vi "UHR-Fleezers Control (host) -Leonardo 04-2018 V3_greenctrl.vi"(0 "Tab Green FB":T5(tab)=enum."Trap Control (RF)") -> ()   [LabVIEW 2013] (continued)
  n84 = property on="2D or 1D Scan" class="Bool (strict)"("Val(Sgnl)"=w155) -> ()  [unwired: 2 in, 2 out]
  n85 = xnode "Read/Write Control"("FPGA VI Reference In"=w152, "error in"=w172, "ai count"="AI Count (ticks)", "Interlace ON/OFF"=w138, "Number Interlace Cycles"=w137, "Set 1"=w18, "Set 2"=w17, "Set 3"=w16, "FB On/Off Set 1"=w259, "FB On/Off Set 2"=w258, "Interlace Off Parameters"=w136, "FB Setpoint Set 1"=w250, "FB Setpoint Set 2"=w249, "FB Gains"="PID gains", "FB output range"=cluster{"output high":i16, "output low":i16} {"output high"=3000, "output low"=0} ("FB output range 1"), "Cycles per step"=w235, "Scan BD"=w247, "Number of scans"=w231, "Scan steps"=w236, "Scan freq.  increment"=w237, "AO1 (Y)"=w219, "AO2 (X)"=w218, "Scan freq.  increment (MCL)"=w212, "Scan steps (MCL)"=w211, "Cycles per step (MCL)"=w210, "Number of scans (MCL)"=w209, "MCL count"=w135, "Cont. Scan (MCL)"=w208, "MCL Scan Axis"=w202, "1D or 2D Scan?"=w155, "N of AI1 Int Acq Sets"=w192, "BD 1 Delay (ticks)"="Freq switch delay", "Amp switch delay"="Amp switch delay", "Swap F1 and F2"="Swap F1 and F2", "APD Acq Rate Count"=w160, "APD to FIFO"=FALSE, "APD Gate Operating Mode"="APD Gate", "APD Gate ON Count"="APD Gate ON Count", "APD Gate OFF Count"="APD Gate OFF Count", "Invert APD Gate"="Invert APD Gate", "DIO count 1 (ticks)"="DIO count 1 (ticks)", "DIO count 2 (ticks)"="DIO count 2 (ticks)", "DIO count 3 (ticks)"="DIO count 3 (ticks)", "APD 1 AO scale factor"="APD 1 AO Mult.", "APD 2 AO scale factor"="APD 2 AO Mult.", "Diff FB Measurement?"=w23, "Dynamic Force FB (Ronen)"=w22, "Negate Diff?"=w21, "Next trap write delay (ticks)"="Next trap write delay (ticks)", "Phase offset method"="Phase offset method", "Phase Trap 1"="Phase increment trap 1", "RF phase reset before cycles"="RF phase reset before cycles", "Phase Trap 2"="Phase increment trap 2") -> ("FPGA VI Reference Out"=w130:T20, "error out"=w132:errorcluster)  [unwired: 1 in]
  n86 = local read "Green Laser ON/Interlacing"() -> (w133:bool)
  n87 = local read "Green laser mode"() -> (w134:enum32{"Laser ON", "Laser OFF", "Interlace"})
  n88 = local read "GI Frequency, OFF count"() -> (w126:u32)
  n89 = local read "GI Frequency, ON count"() -> (w125:u32)
  n90 = Multiply(x="Current When FB OFF (%)", y=655.35) -> (x*y=w116:dbl)
  n91 = local read "Green FB Count"() -> (w124:u32)
  n92 = Multiply(x="Green FB Setpoint (mV)", y=3.2767) -> (x*y=w113:dbl)
  n93 = To Unsigned Word Integer(number=w116) -> (unsigned 16bit integer=w114:u16)
  n94 = local read "Invert GI"() -> (w128:bool)
  n95 = To Word Integer(number=w113) -> (16bit integer=w111:i16)
  n96 = case shown="True" w133 {
    tunnel: w134 -> [_ w294]
    tunnel: [enum32{"Laser ON", "Laser OFF", "Interlace"}."Laser OFF" ("Green laser mode") w294] -> w127
    frame False {
    }
    frame True {
    }
  }
  n97 = local read "Trap Pos. AI1 X Pre-scale"() -> (w82:u16)
  n98 = local read "Trap Pos FB Monitor\nT1 or T2"() -> (w89:bool)
  n99 = local read "Trap Pos FB Int Count"() -> (w79:u16)
  n100 = local read "Trap Pos FB Negate Action"() -> (w88:bool)
  n101 = local read "Trap Pos. FB Offset Factor"() -> (w87:i64)
  n102 = local read "Trap Pos. FB Mult Factor"() -> (w86:i64)
  n103 = local read "Trap Pos. FB Gains"() -> (w84:T11)
  n104 = local read "Trap Pos. FB Range"() -> (w85:T12)
  n105 = xnode "Read/Write Control"("FPGA VI Reference In"=w130, "error in"=w132, "Green interlace ON count 2"=w125, "Green interlace OFF count 2"=w126, "Invert GI 2"=w128, "Operating Mode 2"=w127, "Green FB Gains"="Green FB Gains", "Green FB Setpoint"=w111, "Green FB On/Off"="Green FB On/Off", "Current Out"=w114, "Green int current ON count adj"="Green int current ON count adj", "Green FB Count"=w124, "Operating Mode"=w127, "Green interlace OFF count"=w126, "Green interlace ON count"=w125, "Invert GI"=w128, "Trap Pos FB Monitor T1 or T2"=w89, "Trap Pos FB Negate Action"=w88, "Trap Pos. FB Offset Factor"=w87, "Trap Pos. FB Mult Factor"=w86, "Trap pos. FB Range"=w85, "Trap Pos. FB Gains"=w84, "Force feedback"=FALSE, "AI1 X Scale"=w82, "Trap Pos to FIFO"=TRUE, "Trap Pos FB Int Count"=w79) -> ("FPGA VI Reference Out"=w129:T20, "error out"=w131:errorcluster)
  n106 = xnode "Invoke Method"("FPGA VI Reference In"=w129, "error in"=w131, "Requested Depth"="Trap AI FIFO Depth") -> ("FPGA VI Reference Out"=w92:T20, "error out"=w91:errorcluster)  [unwired: 1 out]
  n107 = xnode "Invoke Method"("FPGA VI Reference In"=w92, "error in"=w91, "Requested Depth"="Trap Position FIFO Depth") -> ("FPGA VI Reference Out"=w6:T20, "error out"=w4:errorcluster)  [unwired: 1 out]
  n108 = xnode "Invoke Method"("FPGA VI Reference In"=w6, "error in"=w4, "Requested Depth"="APD FIFO Depth (requires restart)") -> ("FPGA VI Reference Out"=w5:T20, "error out"=w3:errorcluster)  [unwired: 1 out]
  n109 = flat-sequence {
    tunnel: w153 -> [w299]
    tunnel: [w299] -> w152
    tunnel: [w295] -> w39
    tunnel: [w298] -> w151
    tunnel: [w297] -> w149
    tunnel: [w296] -> w150
    frame #0 {
      w296 = T16 {"Minimum"=60.0, "Maximum"=90.0, "Increment"=1.0} ("Min Max Inc")
      w297 = T16 {"Minimum"=0.0, "Maximum"=75.0, "Increment"=1.0} ("Data Entry Limits")
      w295 = T16 {"Minimum"=60.0, "Maximum"=90.0, "Increment"=1.0} ("Min Max Inc")
      w298 = T16 {"Minimum"=0.0, "Maximum"=75.0, "Increment"=1.0} ("Data Entry Limits")
      n110 = property on="BD 2 Frequency 1 (MHz)" class="DigNum (strict)"("Data Range"=w296) -> ()  [unwired: 2 in, 2 out]
      n111 = property on="BD 2 Frequency 3 (MHz)" class="DigNum (strict)"("Data Range"=w296) -> ()  [unwired: 2 in, 2 out]
      n112 = property on="BD 2 Frequency 2 (MHz)" class="DigNum (strict)"("Data Range"=w296) -> ()  [unwired: 2 in, 2 out]
      n113 = property on="BD 1 Frequency 1 (MHz)" class="DigNum (strict)"("Data Range"=w295) -> ()  [unwired: 2 in, 2 out]
      n114 = property on="BD 1 Frequency 2 (MHz)" class="DigNum (strict)"("Data Range"=w295) -> ()  [unwired: 2 in, 2 out]
      n115 = property on="BD 1 Frequency 3 (MHz)" class="DigNum (strict)"("Data Range"=w295) -> ()  [unwired: 2 in, 2 out]
      n116 = property on="BD 2 Amplitude 1 (%)" class="DigNum (strict)"("Data Range"=w297) -> ()  [unwired: 2 in, 2 out]
      n117 = property on="BD 2 Amplitude 2 (%)" class="DigNum (strict)"("Data Range"=w297) -> ()  [unwired: 2 in, 2 out]
      n118 = property on="BD 2 Amplitude 3 (%)" class="DigNum (strict)"("Data Range"=w297) -> ()  [unwired: 2 in, 2 out]
      n119 = property on="BD 1 Amplitude 3 (%)" class="DigNum (strict)"("Data Range"=w298) -> ()  [unwired: 2 in, 2 out]
      n120 = property on="BD 1 Amplitude 2 (%)" class="DigNum (strict)"("Data Range"=w298) -> ()  [unwired: 2 in, 2 out]
      n121 = property on="BD 1 Amplitude 1 (%)" class="DigNum (strict)"("Data Range"=w298) -> ()  [unwired: 2 in, 2 out]
      "X RF Frequency Limits (MHz)" <- w295
      "X RF Amplitude Limits (%)" <- w298
      "Y RF Amplitude Limits (%)" <- w297
      "Y RF Frequency Limits (MHz)" <- w296
    }
  }
  n122 = xnode "Invoke Method"("FPGA VI Reference In"=w5, "error in"=w3) -> ("FPGA VI Reference Out"=w59:T20, "error out"=w58:errorcluster)  [unwired: 1 in]
  n123 = flat-sequence "Initial FPGA Loop Relative Phase Adjustment" {
    tunnel: "Initial Phase Adjustment (APD 2 Gate)" -> [w301]
    tunnel: "Initial Phase Adjustment (GI) 2" -> [w302]
    tunnel: "Initial Phase Adj. (MCL)" -> [w303]
    tunnel: w58 -> [w304]
    tunnel: w59 -> [w305]
    tunnel: "Initial Phase Adjustment (GI)" -> [w306]
    tunnel: "Initial Phase Adjustment (AI1)" -> [w307]
    tunnel: [w307] -> w68
    tunnel: [w306] -> w67
    tunnel: [w305] -> w66
    tunnel: [w304] -> w65
    tunnel: [w303] -> w64
    tunnel: [w302] -> w63
    tunnel: [w301] -> w62
    tunnel: [w319] -> w178
    tunnel: [w313] -> w176
    tunnel: "Initial Phase Adjustment (APD Acq)" -> [w312]
    tunnel: "Initial Phase Adjustment (APD 1 Gate)" -> [w311]
    tunnel: "Initial Phase Adjustment (Green FB)" -> [w310]
    tunnel: w68 -> [w318]
    tunnel: w67 -> [w317]
    tunnel: w66 -> [w316]
    tunnel: w65 -> [w315]
    tunnel: w64 -> [w314]
    tunnel: w63 -> [w309]
    tunnel: w62 -> [w308]
    tunnel: w178 -> [w321]
    tunnel: [w322] -> w177
    tunnel: w176 -> [w322]
    tunnel: [w321] -> w175
    tunnel: w177 -> [w325]
    tunnel: w175 -> [w324]
    tunnel: [w327] -> w174
    tunnel: [w326] -> w173
    tunnel: [w329] -> w57
    tunnel: [w330] -> w60
    tunnel: w174 -> [w330]
    tunnel: w173 -> [w329]
    frame #0 {
      n124 = Wait (ms)(milliseconds to wait=u32 1000) -> ()  [unwired: 1 out]
    }
    frame #1 {
      n125 = xnode "Read/Write Control"("FPGA VI Reference In"=w316, "error in"=w315, "Phase count adjustment"=w318, "Phase count adjustment (GI)"=w317, "Phase count adjustment (MCL)"=w314, "Phase Count Adjustment (APD Acq)"=w312, "Phase count adjustment (APD 1 Gate)"=w311, "Phase count adjustment (APD 2 Gate)"=w308, "Phase count adjustment (Green FB)"=w310, "Phase count adjustment (GI) 2"=w309) -> ("FPGA VI Reference Out"=w313:T20, "error out"=w319:errorcluster)
    }
    frame #2 {
      n126 = Wait (ms)(milliseconds to wait=u32 1000) -> ()  [unwired: 1 out]
    }
    frame #3 {
      w323 = TRUE
      n127 = xnode "Read/Write Control"("FPGA VI Reference In"=w325, "error in"=w324, "+ phase"=w323, "+ phase (GI)"=w323, "+ phase (MCL)"=w323, "+ phase (APD Acq)"=w323, "+ phase (APD 1 Gate)"=w323, "+ phase (APD 2 Gate)"=w323, "+ phase (Green FB)"=w323, "+ phase (GI) 2"=w323) -> ("FPGA VI Reference Out"=w326:T20, "error out"=w327:errorcluster)
    }
    frame #4 {
      n128 = Wait (ms)(milliseconds to wait=u32 1000) -> ()  [unwired: 1 out]
    }
  }
  n129 = Unbundle By Name(w39) -> ("Minimum"=w38:dbl, "Maximum"=w37:dbl)
  n130 = local read "Phase adj. (Green FB)"() -> (w147:i16)
  n131 = local read "Phase adj. (GI) 2"() -> (w117:i16)
  n132 = local read "Phase adjust (MCL)"() -> (w203:i16)
  n133 = local read "Phase adj. (AI1)"() -> (w205:i16)
  n134 = local read "Phase adj. (GI)"() -> (w204:i16)
  n135 = Multiply(x=w38, y=w36) -> (x*y=w34:dbl)
  n136 = Multiply(x=w37, y=w36) -> (x*y=w35:dbl)
  n137 = Multiply(x=49152000.0, y=6.0) -> (x*y=w28:dbl)
  n138 = Scale By Power Of 2(n=w33, x=w34) -> (x*2^n=w30:dbl)
  n139 = Scale By Power Of 2(n=w33, x=w35) -> (x*2^n=w29:dbl)
  n140 = xnode "Read/Write Control"("FPGA VI Reference In"=w57, "error in"=w60, "Phase count adjustment"=w205, "Phase count adjustment (GI)"=w204, "Phase count adjustment (MCL)"=w203, "Phase Count Adjustment (APD Acq)"="Phase Adj. (APD Acq)", "Phase count adjustment (APD 1 Gate)"="Phase Adj. (APD 1 Gate)", "Phase count adjustment (APD 2 Gate)"="Phase Adj. (APD 2 Gate)", "Phase count adjustment (Green FB)"=w147, "Phase count adjustment (GI) 2"=w117) -> ("FPGA VI Reference Out"=w14:T20, "error out"=w13:errorcluster)
  n141 = Divide(x=w29, y=w28) -> (x/y=w26:dbl)
  n142 = Divide(x=w30, y=w28) -> (x/y=w27:dbl)
  n143 = To Unsigned Quad Integer(1:w27) -> (0:w25:u64)
  n144 = To Unsigned Quad Integer(1:w26) -> (0:w24:u64)
  n145 = xnode "Read/Write Control"("FPGA VI Reference In"=w14, "FB Min frequency"=w25, "FB Max Frequency"=w24) -> ()  [unwired: 1 in, 2 out]
  n146 = call "set RF board frequency - interlace.vi"("Board 2 Frequency Limits"=w150, "Board 1 Frequency Limits"=w39, "error in"=w13, "FPGA VI Reference In"=w14, "Board 2 Frequency 3 (MHz)"="BD 2 Frequency 3 (MHz)", "Board 1 Frequency 3 (MHz)"="BD 1 Frequency 3 (MHz)", "Board 2 Frequency 2 (MHz)"="BD 2 Frequency 2 (MHz)", "Board 2 Frequency 1 (MHz)"="BD 2 Frequency 1 (MHz)", "Board 1 Frequency 2 (MHz)"="BD 1 Frequency 2 (MHz)", "Board 1 Frequency 1  (MHz)"="BD 1 Frequency 1 (MHz)") -> ("error out"=w270:errorcluster, "FPGA VI Reference Out"=w271:T20)
  n147 = call "set RF board amplitude - interlace.vi"("Board 2 Amplitude Limits"=w149, "Board 1 Amplitude Limits"=w151, "error in"=w270, "FPGA VI Reference In"=w271, "Board 2 Amplitude 3 (%)"="BD 2 Amplitude 3 (%)", "Board 1 Amplitude 3 (%)"="BD 1 Amplitude 3 (%)", "Board 2 Amplitude 2 (%)"="BD 2 Amplitude 2 (%)", "Board 2 Amplitude 1 (%)"="BD 2 Amplitude 1 (%)", "Board 1 Amplitude 2 (%)"="BD 1 Amplitude 2 (%)", "Board 1 Amplitude 1 (%)"="BD 1 Amplitude 1 (%)") -> ("error out"=w55:errorcluster, "FPGA VI Reference Out"=w56:T20)
  n148 = flat-sequence {
    tunnel: w56 -> [w332]
    tunnel: w55 -> [w331]
    tunnel: [w332] -> w263
    tunnel: [w331] -> w262
    tunnel: [w340] -> w261
    tunnel: w263 -> [w340]
    tunnel: [w339] -> w260
    tunnel: w262 -> [w339]
    tunnel: w261 -> [w343]
    tunnel: w260 -> [w342]
    tunnel: [w343] -> w51
    tunnel: [w342] -> w50
    tunnel: [w349] -> w76
    tunnel: [w353] -> w61
    tunnel: w51 -> [w353]
    tunnel: w50 -> [w348]
    frame #0 {
      n149 = local read "Trap 1 (ON/OFF)"() -> (w333:bool)
      n150 = local write "Saving..."(FALSE ("Saving Data")) -> ()
      n151 = local write "Stop All"(FALSE ("Stop All")) -> ()
      n152 = local write "Index"(1.0 ("Index")) -> ()
      n153 = property on="Trap 1 ON" class="Bool (strict)"("Value"=w333) -> ()  [unwired: 2 in, 2 out]
      "Manipulating Trap" <- FALSE ("Manipulating Trap")
    }
    frame #1 {
      n154 = local read "Trap 2 (ON/OFF)"() -> (w338:bool)
      n155 = Wait (ms)(milliseconds to wait=u32 50) -> ()  [unwired: 1 out]
      n156 = property on="Trap 2 ON" class="Bool (strict)"("Val(Sgnl)"=w338) -> ()  [unwired: 2 in, 2 out]
    }
    frame #2 {
      n157 = local read "Scan Range (nm)"() -> (w344:dbl)
      n158 = call "Update messages.vi"("Message to add"="UHR-Fleezers ready.", "Old message string"="") -> ("New message string"=w347:string)
      n159 = local write "Messages"(w347) -> ()
      n160 = property on="Scan Range (nm)" class="DigNum (strict)"("Val(Sgnl)"=w344) -> ()  [unwired: 2 in, 2 out]
    }
    frame #3 {
      n161 = call "hamilton_controller.vi"("error in"=w348, "action"=T21."CONNECT") -> ("error out"=w350:errorcluster)  [unwired: 9 in]
      n162 = call "hamilton_controller.vi"("error in"=w350, "action"=T21."INITIALIZE VALVES") -> ("error out"=w349:errorcluster)  [unwired: 9 in]
    }
  }
  n163 = Subtract(x="BD 1 Frequency 1 (MHz)", y="BD 1 Frequency 2 (MHz)") -> (x-y=w191:dbl)
  n164 = Subtract(x="BD 2 Frequency 1 (MHz)", y="BD 2 Frequency 2 (MHz)") -> (x-y=w190:dbl)
  n165 = Square(x=w190) -> (x^2=w188:dbl)
  n166 = Square(x=w191) -> (x^2=w189:dbl)
  n167 = Add(x=w189, y=w188) -> (x+y=w187:dbl)
  n168 = Square Root(x=w187) -> (sqrt(x)=w186:dbl)
  n169 = local write "Trap Delta (MHz)"(w186) -> ()
  n170 = call "IMAQ Create"("Image Name"="APD 1 Image", "Image Type"=w98) -> ("New Image"=w97:T3)  [unwired: 3 in, 1 out]
  n171 = call "IMAQ Create"("Image Name"="APD 2 Image", "Image Type"=w98) -> ("New Image"=w96:T3)  [unwired: 3 in, 1 out]
  n172 = call "IMAQ Create"("Image Name"="Det. X Image", "Image Type"=w98) -> ("New Image"=w95:T3)  [unwired: 3 in, 1 out]
  n173 = call "IMAQ Create"("Image Name"="Det. Y Image", "Image Type"=w98) -> ("New Image"=w94:T3)  [unwired: 3 in, 1 out]
  n174 = Bundle("New Image"=w97, "New Image"=w96, "New Image"=w95, "New Image"=w94) -> (w93:T22)  [unwired: 1 in]
  n175 = Current VI's Path() -> (path=w40:path)
  n176 = Concatenate Strings("N.D.", "\r\n") -> (w44:string)
  n177 = Strip Path(path=w40) -> (stripped path=w41:path)  [unwired: 1 out]
  n178 = Initialize Array(w44, 4, 3) -> (w47:string[][])
  n179 = Build Path(base path=w41, name or relative path="Locations.txt") -> (appended path=→"Location path":path)
  n180 = local write "Location Matrix"(w47) -> ()
  n181 = while {
    stop <- w354 stop-if-true
    n182 = event shown="[0] Timeout" {
      selector: _ -> [_ _ _ _ _ _ _ _ _]
      dyn-events: _ -> [_ _ _ _ _ _ _ _ _]
      timeout: 10 -> [_ _ _ _ _ _ _ _ _]
      tunnel: [FALSE _ _ _ _ _ _ _ TRUE] -> w354
      event Timeout {
        # "Change the trajectory mode to Jog"
        # "Query and display stage positions"
        # "Setting ESP300 left and right limits for Z-axis, input in mm"
        # "Display Selected Location"
        n183 = event-data() -> ()  [unwired: 1 in, 2 out]
        n184 = local read "Capture Locations"() -> (w379:i32)
        n185 = local read "Location Matrix"() -> (w380:string[][])
        n186 = Concatenate Strings("1TP;\n2TP;\n3TP;\n1MD?;\n2MD?;\n3MD?" ("Substring"), "\r") -> (w363:string)
        n187 = local read "ESP Port"() -> (w366:refnum<visa-resource-name>)
        n188 = Index Array(array=w380, index (row)=w379) -> (element=w378:string[])  [unwired: 1 in]
        n189 = local read "ESP Port"() -> (w375:refnum<visa-resource-name>)
        n190 = VISA Write(VISA resource name=w366, write buffer=w363, error in (no error)="error in") -> (VISA resource name out=w364:refnum<visa-resource-name>, error out=w362:errorcluster)  [unwired: 1 out]
        n191 = Concatenate Strings("3SL" ("Substring"), "ESP ZL-Limit", ";3SR", "ESP ZR-Limit", "\r") -> (w374:string)
        n192 = Array To Cluster(array=w378) -> (cluster=w377:T23)
        n193 = case shown="True" TRUE ("Case Constant\n(See Context Help)") {
          tunnel: w364 -> [_ w418]
          tunnel: w362 -> [w399 w417]
          tunnel: [w399 w401] -> w368
          frame False {
          }
          frame True {
            w411 = u16 10 items=["1.0"=10, "1.5"=15, "2.0"=20] ("Serial Settings:Stop Bits")
            w412 = u16 0 items=["None", "Odd", "Even", "Mark", "Space"] ("Serial Settings:Parity")
            n194 = property class="Instr"(reference=w418, error in=w417, "Baud"=u32 921600 ("Serial Settings:Baud Rate"), "Data Bits"=u16 8 ("Serial Settings:Data Bits"), "Parity"=w412, "Stop Bits"=w411) -> (reference out=w416:refnum<visa-resource-name>, error out=w415:errorcluster, "Bytes at Port"=w400:u32)
            n195 = Wait (ms)(milliseconds to wait=u32 10) -> ()  [unwired: 1 out]
            n196 = VISA Read(VISA resource name=w416, byte count=w400, error in (no error)=w415) -> (VISA resource name out=w424:refnum<visa-resource-name>, read buffer=→"X Pos":string, error out=w425:errorcluster)  [unwired: 1 out]
            n197 = VISA Read(VISA resource name=w424, byte count=w400, error in (no error)=w425) -> (VISA resource name out=w422:refnum<visa-resource-name>, read buffer=→"Y Pos":string, error out=w423:errorcluster)  [unwired: 1 out]
            n198 = VISA Read(VISA resource name=w422, byte count=w400, error in (no error)=w423) -> (VISA resource name out=w410:refnum<visa-resource-name>, read buffer=→"Z Pos Pos":string, error out=w409:errorcluster)  [unwired: 1 out]
            n199 = VISA Read(VISA resource name=w410, byte count=w400, error in (no error)=w409) -> (VISA resource name out=w406:refnum<visa-resource-name>, read buffer=→"X Motion":string, error out=w407:errorcluster)  [unwired: 1 out]
            n200 = VISA Read(VISA resource name=w406, byte count=w400, error in (no error)=w407) -> (VISA resource name out=w405:refnum<visa-resource-name>, read buffer=→"Y Motion":string, error out=w403:errorcluster)  [unwired: 1 out]
            n201 = VISA Read(VISA resource name=w405, byte count=w400, error in (no error)=w403) -> (read buffer=→"Z motion":string, error out=w401:errorcluster)  [unwired: 2 out]
          }
        }
        "error out" <- w368
        n202 = VISA Write(VISA resource name=w375, write buffer=w374) -> ()  [unwired: 1 in, 3 out]
        n203 = local write item#483(w377) -> ()
        n204 = disable-structure shown="Disabled" {
          frame Disabled {
            # "Change Low Jog Velocity"
            # "Change High Jog Velocity"
            n205 = Concatenate Strings("1JH" ("Substring"), "Axis 1", "2JH" ("Substring"), "Axis 2", "3JH" ("Substring"), "Axis 3", "\r") -> (w398:string)
            n206 = local read "ESP Port"() -> (w397:refnum<visa-resource-name>)
            n207 = VISA Write(VISA resource name=w397, write buffer=w398) -> ()  [unwired: 1 in, 3 out]
            n208 = Concatenate Strings("1JW" ("Substring"), "Axis 1", "2JW" ("Substring"), "Axis 2", "3JW" ("Substring"), "Axis 3", "\r") -> (w389:string)
            n209 = local read "ESP Port"() -> (w388:refnum<visa-resource-name>)
            n210 = VISA Write(VISA resource name=w388, write buffer=w389) -> ()  [unwired: 1 in, 3 out]
          }
          frame Enabled {
          }
        }
        n211 = local read "ESP Port"() -> (w356:refnum<visa-resource-name>)
        n212 = Concatenate Strings("1TJ3;\n2TJ3;\n3TJ3" ("Substring"), "\r") -> (w357:string)
        n213 = VISA Write(VISA resource name=w356, write buffer=w357) -> ()  [unwired: 1 in, 3 out]
      }
      event "Goto Top (F6)": Value Change {
        n214 = event-data() -> ()  [unwired: 1 in, 5 out]
        n215 = stacked-sequence {
          frame #0 {
            # "stop motions of all axes before going to avoid reversing of direction"
            n216 = local read "ESP Port"() -> (w430:refnum<visa-resource-name>)
            n217 = Concatenate Strings("ST" ("Substring"), "\r") -> (w427:string)
            n218 = VISA Write(VISA resource name=w430, write buffer=w427) -> ()  [unwired: 1 in, 3 out]
          }
          frame #1 {
            n219 = Wait (ms)(milliseconds to wait=u32 50) -> ()  [unwired: 1 out]
          }
          frame #2 {
            # "Change the trajectory mode to Trapezoidal"
            n220 = local read "ESP Port"() -> (w435:refnum<visa-resource-name>)
            n221 = Concatenate Strings("1TJ1;\n2TJ1;\n3TJ1" ("Substring"), "\r") -> (w432:string)
            n222 = VISA Write(VISA resource name=w435, write buffer=w432) -> ()  [unwired: 1 in, 3 out]
          }
          frame #3 {
            # "Go to Top Dispensor"
            n223 = local read "Location Matrix"() -> (w447:string[][])
            n224 = Index Array(array=w447, index (row)=0) -> (element=w443:string[])  [unwired: 1 in]
            n225 = Decimate 1D Array(w443) -> (w441:string[], w439:string[], w437:string[])
            n226 = local read "ESP Port"() -> (w444:refnum<visa-resource-name>)
            n227 = Concatenate Strings("1PA" ("Substring"), w441, "2PA" ("Substring"), w439, "3PA" ("Substring"), w437, "\r") -> (w445:string)
            n228 = VISA Write(VISA resource name=w444, write buffer=w445) -> ()  [unwired: 1 in, 3 out]
          }
          frame #4 {
            n229 = Wait (ms)(milliseconds to wait=u32 100) -> ()  [unwired: 1 out]
          }
          frame #5 {
            # "Change the trajectory mode to Jog"
            n230 = local read "ESP Port"() -> (w452:refnum<visa-resource-name>)
            n231 = Concatenate Strings("1TJ3;\n2TJ3;\n3TJ3" ("Substring"), "\r") -> (w449:string)
            n232 = VISA Write(VISA resource name=w452, write buffer=w449) -> ()  [unwired: 1 in, 3 out]
          }
        }
      }
      event "Goto Exp (F8)": Value Change {
        n233 = event-data() -> ()  [unwired: 1 in, 5 out]
        n234 = stacked-sequence {
          frame #0 {
            # "stop motions of all axes before going to avoid reversing of direction"
            n235 = local read "ESP Port"() -> (w456:refnum<visa-resource-name>)
            n236 = Concatenate Strings("ST" ("Substring"), "\r") -> (w453:string)
            n237 = VISA Write(VISA resource name=w456, write buffer=w453) -> ()  [unwired: 1 in, 3 out]
          }
          frame #1 {
            n238 = Wait (ms)(milliseconds to wait=u32 50) -> ()  [unwired: 1 out]
          }
          frame #2 {
            # "Change the trajectory mode to Trapezoidal"
            n239 = local read "ESP Port"() -> (w461:refnum<visa-resource-name>)
            n240 = Concatenate Strings("1TJ1;\n2TJ1;\n3TJ1" ("Substring"), "\r") -> (w458:string)
            n241 = VISA Write(VISA resource name=w461, write buffer=w458) -> ()  [unwired: 1 in, 3 out]
          }
          frame #3 {
            # "Go to Experimental"
            n242 = local read "Location Matrix"() -> (w473:string[][])
            n243 = Index Array(array=w473, index (row)=2) -> (element=w469:string[])  [unwired: 1 in]
            n244 = Decimate 1D Array(w469) -> (w467:string[], w465:string[], w463:string[])
            n245 = Concatenate Strings("1PA" ("Substring"), w467, "2PA" ("Substring"), w465, "3PA" ("Substring"), w463, "\r") -> (w471:string)
            n246 = local read "ESP Port"() -> (w470:refnum<visa-resource-name>)
            n247 = VISA Write(VISA resource name=w470, write buffer=w471) -> ()  [unwired: 1 in, 3 out]
          }
          frame #4 {
            n248 = Wait (ms)(milliseconds to wait=u32 200) -> ()  [unwired: 1 out]
          }
          frame #5 {
            # "Change the trajectory mode to Jog"
            n249 = local read "ESP Port"() -> (w475:refnum<visa-resource-name>)
            n250 = Concatenate Strings("1TJ3;\n2TJ3;\n3TJ3" ("Substring"), "\r") -> (w478:string)
            n251 = VISA Write(VISA resource name=w475, write buffer=w478) -> ()  [unwired: 1 in, 3 out]
          }
        }
      }
      event "Goto Bottom (F7)": Value Change {
        n252 = event-data() -> ()  [unwired: 1 in, 5 out]
        n253 = stacked-sequence {
          frame #0 {
            # "stop motions of all axes before going to avoid reversing of direction"
            n254 = local read "ESP Port"() -> (w482:refnum<visa-resource-name>)
            n255 = Concatenate Strings("ST" ("Substring"), "\r") -> (w479:string)
            n256 = VISA Write(VISA resource name=w482, write buffer=w479) -> ()  [unwired: 1 in, 3 out]
          }
          frame #1 {
            n257 = Wait (ms)(milliseconds to wait=u32 50) -> ()  [unwired: 1 out]
          }
          frame #2 {
            # "Change the trajectory mode to Trapezoidal"
            n258 = local read "ESP Port"() -> (w487:refnum<visa-resource-name>)
            n259 = Concatenate Strings("1TJ1;\n2TJ1;\n3TJ1" ("Substring"), "\r") -> (w484:string)
            n260 = VISA Write(VISA resource name=w487, write buffer=w484) -> ()  [unwired: 1 in, 3 out]
          }
          frame #3 {
            # "Go to Bottom Dispensor"
            n261 = local read "Location Matrix"() -> (w499:string[][])
            n262 = Index Array(array=w499, index (row)=1) -> (element=w495:string[])  [unwired: 1 in]
            n263 = Decimate 1D Array(w495) -> (w493:string[], w491:string[], w489:string[])
            n264 = Concatenate Strings("1PA" ("Substring"), w493, "2PA" ("Substring"), w491, "3PA" ("Substring"), w489, "\r") -> (w497:string)
            n265 = local read "ESP Port"() -> (w496:refnum<visa-resource-name>)
            n266 = VISA Write(VISA resource name=w496, write buffer=w497) -> ()  [unwired: 1 in, 3 out]
          }
          frame #4 {
            n267 = Wait (ms)(milliseconds to wait=u32 200) -> ()  [unwired: 1 out]
          }
          frame #5 {
            # "Change the trajectory mode to Jog"
            n268 = local read "ESP Port"() -> (w501:refnum<visa-resource-name>)
            n269 = Concatenate Strings("1TJ3;\n2TJ3;\n3TJ3" ("Substring"), "\r") -> (w504:string)
            n270 = VISA Write(VISA resource name=w501, write buffer=w504) -> ()  [unwired: 1 in, 3 out]
          }
        }
      }
      event "Capture": Value Change {
        n271 = event-data() -> ()  [unwired: 1 in, 5 out]
        n272 = local read "Capture Locations"() -> (w505:i32)
        n273 = local read "Z Pos Pos"() -> (w506:string)
        n274 = local read "X Pos"() -> (w508:string)
        n275 = local read "Y Pos"() -> (w507:string)
        n276 = case shown="1" w505 {
          selector: w505 -> [w512 w519 w526 w533]
          tunnel: w508 -> [w515 w522 w529 w536]
          tunnel: w507 -> [w514 w521 w528 w535]
          tunnel: w506 -> [w513 w520 w527 w534]
          frame 0, Default {
            # "Capture Top Dispensor Location"
            n277 = local read "Location Matrix"() -> (w511:string[][])
            n278 = Build Array(w515, w514, w513) -> (w510:string[])
            n279 = Replace Array Subset(array=w511, new element=w510, index (row)=w512) -> (w509:string[][])  [unwired: 1 in]
            n280 = local write "Location Matrix"(w509) -> ()
          }
          frame 1 {
            # "Capture Bottom Dispensor Location"
            n281 = local read "Location Matrix"() -> (w518:string[][])
            n282 = Build Array(w522, w521, w520) -> (w517:string[])
            n283 = Replace Array Subset(array=w518, new element=w517, index (row)=w519) -> (w516:string[][])  [unwired: 1 in]
            n284 = local write "Location Matrix"(w516) -> ()
          }
          frame 2 {
            # "Capture Experimental Region Location"
            n285 = local read "Location Matrix"() -> (w525:string[][])
            n286 = Build Array(w529, w528, w527) -> (w524:string[])
            n287 = Replace Array Subset(array=w525, new element=w524, index (row)=w526) -> (w523:string[][])  [unwired: 1 in]
            n288 = local write "Location Matrix"(w523) -> ()
          }
          frame 3 {
            # "Capture Other Location"
            n289 = local read "Location Matrix"() -> (w532:string[][])
            n290 = Build Array(w536, w535, w534) -> (w531:string[])
            n291 = Replace Array Subset(array=w532, new element=w531, index (row)=w533) -> (w530:string[][])  [unwired: 1 in]
            n292 = local write "Location Matrix"(w530) -> ()
          }
        }
      }
      event "Save": Value Change {
        # "reshape Location Matrix to 1-D array to write"
        n293 = event-data() -> ()  [unwired: 1 in, 5 out]
        n294 = local read "Location Matrix"() -> (w540:string[][])
        n295 = local read "Location path"() -> (w537:path)
        n296 = Reshape Array(w540, 12) -> (w538:string[])
        n297 = Write to Text File(file (use dialog)=w537, text=w538) -> ()  [unwired: 2 in, 3 out]
      }
      event "VISA Clear": Value Change {
        n298 = event-data() -> ()  [unwired: 1 in, 5 out]
        n299 = local read "ESP Port"() -> (w541:refnum<visa-resource-name>)
        n300 = VISA Clear(VISA resource name=w541) -> ()  [unwired: 1 in, 2 out]
      }
      event "Activate Joystick": Value Change {
        # "Change the trajectory mode to Jog"
        n301 = event-data() -> ()  [unwired: 1 in, 5 out]
        n302 = disable-structure shown="Disabled" {
          frame Disabled {
            n303 = case shown="True" "Activate Joystick" {
              frame False {
              }
              frame True {
                # "Change the trajectory mode to Jog"
                n304 = local read "ESP Port"() -> (w550:refnum<visa-resource-name>)
                n305 = Concatenate Strings("1TJ3;\n2TJ3;\n3TJ3" ("Substring"), "\r") -> (w547:string)
                n306 = VISA Write(VISA resource name=w550, write buffer=w547) -> ()  [unwired: 1 in, 3 out]
              }
            }
          }
          frame Enabled {
          }
        }
        n307 = local read "ESP Port"() -> (w542:refnum<visa-resource-name>)
        n308 = Concatenate Strings("1TJ3;\n2TJ3;\n3TJ3" ("Substring"), "\r") -> (w545:string)
        n309 = VISA Write(VISA resource name=w542, write buffer=w545) -> ()  [unwired: 1 in, 3 out]
      }
      event "Stop All": Mouse Down {
        n310 = event-data() -> ()  [unwired: 1 in, 5 out]
      }
    }
  }
  n311 = disable-structure shown="Disabled" {
    disable-tunnel: w61 -> [w580 _]
    frame Disabled {
      w575 = T17 0 items=["Grayscale (U8)", "Grayscale (I16)", "Grayscale (SGL)", "Complex (CSG)", "RGB (U32)", "HSL (U32)", "RGB (U64)", "Grayscale (U16)"] ("Image Type")
      n312 = call <vilib>:"IMAQ Init.vi"("Interface Name"="img0") -> ("error out"=w577:errorcluster, "IMAQ Session Out"=w579:refnum<k11>)  [unwired: 9 in]
      n313 = call <vilib>:"IMAQ Grab Setup.vi"("error in (no error)"=w577, "IMAQ Session In"=w579) -> ("error out"=w573:errorcluster, "IMAQ Session Out"=w574:refnum<k11>)  [unwired: 8 in]
      n314 = call "IMAQ Create"("Image Name"="untitled", "Image Type"=w575) -> ("New Image"=w572:T3)  [unwired: 3 in, 1 out]
      n315 = call <vilib>:"Application Directory.vi"() -> ("Application Directory"=w559:path)
      n316 = Build Path(base path=w559, name or relative path="_trap_screen_positions") -> (appended path=w567:path)
      n317 = Open/Create/Replace File(file path (use dialog)=w567, operation (0:open)=T24."open or create", access (0:read/write)=enum16{"read/write", "read-only", "write-only"}."read/write") -> (refnum out=w569:refnum<file>)  [unwired: 3 in, 2 out]
      n318 = local read "Trap Sets"() -> (w561:u32)
      n319 = for "Load trap positions on video screen from file." {
        N: w561 -> [_]
        tunnel: [w587] -> w562
        tunnel: w569 -> [w586]
        tunnel: [w583] -> w558 mode=indexing
        w585 = 4
        n320 = for {
          N: w585 -> [_]
          tunnel: [w591] -> w587
          tunnel: w586 -> [w590]
          tunnel: w585 -> [w589]
          tunnel: [w588] -> w584 mode=indexing
          n321 = Read from Binary File(5:w589, 11:w590) -> (2:w588:i32, 3:w591:refnum<file>)  [unwired: 4 in, 2 out]
        }
        n322 = Array To Cluster(array=w584) -> (cluster=w583:T28)
      }
      n323 = node-c288() -> (w582:T25)  [unwired: 4 in]
      n324 = timed-loop "acquire video and stage position" {
        timing: w582 -> [_]
        timing-out: [_] -> w581
        tunnel: w574 -> [w610]
        tunnel: w573 -> [w609]
        tunnel: w572 -> [w608]
        tunnel: [w607] -> w554
        tunnel: [w604] -> w555
        tunnel: [w605] -> w553
        tunnel: w580 -> [_]
        shift-right: [w601] -> w571
        shift-left: w558 -> [w602]
        tunnel: w561 -> [w599]
        stop <- w606 stop-if-true
        n325 = node-c288() -> ()  [unwired: 1 in, 1 out]
        n326 = event shown="[1] \"Stop All\": Value Change" {
          selector: _ -> [_ _ _ _]
          dyn-events: _ -> [_ _ _ _]
          timeout: 10 -> [_ _ _ _]
          tunnel: w610 -> [w621 w636 w645 w664]
          tunnel: w609 -> [w620 w638 w643 w666]
          tunnel: w608 -> [w619 w637 w644 w665]
          tunnel: [w618 w636 w645 w664] -> w607
          tunnel: [w611 w640 FALSE FALSE] -> w606
          tunnel: [w615 w638 w643 w666] -> w605
          tunnel: [w614 w637 w644 w665] -> w604
          tunnel: "radius" -> [_ _ w650 _]
          tunnel: w602 -> [w612 w639 w648 _]
          tunnel: [w612 w639 w649 cluster{i32, i32, i32, i32}[] []] -> w601
          tunnel: w599 -> [_ _ w641 _]
          event Timeout {
            n327 = event-data() -> ()  [unwired: 1 in, 2 out]
            n328 = call <vilib>:"IMAQ Grab Acquire.vi"("error in (no error)"=w620, "Image In"=w619, "IMAQ Session In"=w621) -> ("error out"=w616:errorcluster, "Image Out"=w617:T3, "IMAQ Session Out"=w618:refnum<k11>)  [unwired: 5 in, 1 out]
            n329 = case shown="True" "trap\nmarkers?" {
              tunnel: w612 -> [_ w629]
              tunnel: w617 -> [w623 w628]
              tunnel: w616 -> [w622 w627]
              tunnel: [w622 w626] -> w615
              tunnel: [w623 w624] -> w614
              frame False {
              }
              frame True {
                n330 = for {
                  tunnel: w629 -> [w635] mode=indexing
                  shift-right: [w633] -> w624
                  shift-left: w628 -> [w634]
                  tunnel: w627 -> [w632]
                  tunnel: [w631] -> w626
                  tunnel: u32 16711680 ("Color") -> [w630]
                  n331 = call "IMAQ Overlay Oval"("Color"=w630, "error in (no error)"=w632, "Bounding Rectangle"=w635, "Image"=w634) -> ("error out"=w631:errorcluster, "Image Out"=w633:T3)  [unwired: 6 in]
                }
              }
            }
            "Primary Video Display" <- w614
            n332 = Unbundle By Name(w616) -> ("status"=w611:bool)
          }
          event "Stop All": Value Change {
            n333 = event-data() -> ()  [unwired: 1 in, 5 out]
            n334 = local read "Stop All"() -> (w640:bool)
          }
          event "Primary Video Display": Mouse Down {
            n335 = event-data() -> ()  [unwired: 1 in, 7 out]
            n336 = Array Size(array=w648) -> (size(s)=w647:i32)
            n337 = Less?(x=w647, y=w641) -> (x < y?=w646:bool)
            n338 = case shown="True" w646 {
              tunnel: w650 -> [_ w660]
              tunnel: w648 -> [w651 w654]
              tunnel: [w651 w653] -> w649
              frame False {
              }
              frame True {
                n339 = property on="Primary Video Display" class="ImageControl"() -> ("Last Mouse Position"=w652:cluster{"X":i32, "Y":i32})  [unwired: 2 in, 2 out]
                n340 = Unbundle By Name(w652) -> ("X"=w662:i32, "Y"=w661:i32)
                n341 = Add(x=w661, y=w660) -> (x+y=w658:i32)
                n342 = Subtract(x=w661, y=w660) -> (x-y=w656:i32)
                n343 = Add(x=w662, y=w660) -> (x+y=w657:i32)
                n344 = Subtract(x=w662, y=w660) -> (x-y=w659:i32)
                n345 = Bundle(w659, w658, w657, w656) -> (w655:cluster{i32, i32, i32, i32})  [unwired: 1 in]
                n346 = Build Array (concatenate)(w654, w655) -> (w653:T29)
              }
            }
          }
          event "clear markers": Value Change {
            n347 = event-data() -> ()  [unwired: 1 in, 5 out]
          }
        }
        n348 = node-c288() -> ()  [unwired: 1 in, 1 out]
      }
      n349 = node-c288(w581) -> ()  [unwired: 1 out]
      n350 = Set File Position(offset (in bytes) (0)=i64 0, refnum=w562, from (0:start)=enum16{"start", "end", "current"}."start") -> (refnum out=w563:refnum<file>)  [unwired: 1 in, 1 out]
      n351 = for "Write trap positions to file so they can be remembered\nwhen program is removed from memory" {
        tunnel: w571 -> [w595] mode=indexing
        tunnel: [w593] -> w570
        tunnel: w563 -> [w592]
        n352 = Cluster To Array(cluster=w595) -> (array=w594:i32[])
        n353 = for {
          tunnel: w594 -> [w598] mode=indexing
          tunnel: [w597] -> w593
          tunnel: w592 -> [w596]
          n354 = Write to Binary File(file (use dialog)=w596, data=w598) -> (refnum out=w597:refnum<file>)  [unwired: 4 in, 2 out]
        }
      }
      n355 = Close File(refnum=w570) -> ()  [unwired: 1 in, 2 out]
      n356 = call "IMAQ Dispose"("Image"=w555, "error in (no error)"=w553) -> ("error out"=w552:errorcluster)  [unwired: 4 in]
      n357 = call <vilib>:"IMAQ Stop.vi"("error in (no error)"=w552, "IMAQ Session In"=w554) -> ("error out"=w556:errorcluster, "IMAQ Session Out"=w557:refnum<k11>)  [unwired: 8 in]
      n358 = call <vilib>:"IMAQ Close.vi"("error in (no error)"=w556, "IMAQ Session In"=w557) -> ()  [unwired: 9 in, 1 out]
    }
    frame Enabled {
    }
  }
  n359 = disable-structure shown="Enabled" {
    disable-tunnel: [w673 _] -> w71
    disable-tunnel: w61 -> [w672 _]
    frame Enabled {
      n360 = node-c288() -> (w675:T25)  [unwired: 4 out]
      n361 = timed-loop "Rough control of MCL mirror stage (debugging)" {
        tunnel: w672 -> [w678]
        tunnel: [w677] -> w673
        timing: w675 -> [_]
        timing-out: [_] -> w674
        stop <- w677 stop-if-true
        n362 = node-c288() -> ()  [unwired: 2 out]
        n363 = case shown="1" "MCL Mode" {
          tunnel: w678 -> [_ w681 w728]
          frame 0, Default {
            # "manual positioning"
          }
          frame 1 {
            # "sinusoidal wave"
            n364 = node-c288() -> (w683:T25)  [unwired: 4 out]
            n365 = timed-loop "Oscillate MCL mirror" {
              timing: w683 -> [_]
              timing-out: [_] -> w682
              tunnel: w681 -> [w722]
              i -> [w721]
              stop <- w684 stop-if-true
              n366 = node-c288() -> (w720:i64)  [unwired: 1 out]
              n367 = Multiply(x="AO1", y=32767.0) -> (x*y=w716:dbl)
              n368 = Multiply(x="AO2", y=32767.0) -> (x*y=w711:dbl)
              n369 = Divide(x=w716, y=10.0) -> (x/y=w717:dbl)
              n370 = Divide(x=w711, y=10.0) -> (x/y=w712:dbl)
              n371 = To Word Integer(number=w717) -> (16bit integer=w709:i16)
              n372 = To Word Integer(number=w712) -> (16bit integer=w708:i16)
              n373 = Divide(x=w720, y=i64 1000) -> (x/y=w691:dbl)
              n374 = Multiply(x=w691, y=w721) -> (x*y=w702:dbl)
              n375 = Multiply(x="Osc. freq. (Hz) 2", y=6.283185307179586) -> (x*y=w703:dbl)
              n376 = Multiply(x=w703, y=w702) -> (x*y=w701:dbl)
              n377 = Sine(x=w701) -> (sin(x)=w700:dbl)
              n378 = Multiply(x=w700, y="Osc. amp. (V)") -> (x*y=w698:dbl)
              n379 = Add(x=w698, y="Osc. center (V)") -> (x+y=w696:dbl)
              n380 = Divide(x=w696, y=10.0) -> (x/y=w694:dbl)
              n381 = Multiply(x=w694, y=32767.0) -> (x*y=w689:dbl)
              n382 = Select(t=w689, s="Scan axis", f=w709) -> (s? t:f=w707:dbl)
              n383 = Select(t=w708, s="Scan axis", f=w689) -> (s? t:f=w706:dbl)
              n384 = local read "MCL Mode"() -> (w688:u16)
              n385 = Not Equal?(x=w688, y=u16 1) -> (x != y?=w685:bool)
              n386 = local read "Stop All"() -> (w686:bool)
              n387 = xnode "Read/Write Control"("FPGA VI Reference In"=w722, "AO1 (Y)"=w707, "AO2 (X)"=w706) -> ()  [unwired: 1 in, 2 out]
              n388 = Compound Arithmetic op=OR(w686, w685) -> (w684:bool)
              n389 = node-c288() -> ()  [unwired: 2 out]
            }
            n390 = node-c288(w682) -> ()  [unwired: 1 out]
          }
          frame 2 {
            # "linear scan"
            n391 = case shown="True" "Start Scan" {
              tunnel: w728 -> [_ w740]
              frame False {
              }
              frame True {
                n392 = Subtract(x="End (V)", y="Begin (V)") -> (x-y=w736:dbl)
                n393 = Decrement(x="N Points") -> (x-1=w735:dbl)
                n394 = Divide(x=w736, y=w735) -> (x/y=w733:dbl)
                n395 = for {
                  N: "N Points" -> [_]
                  tunnel: "Begin (V)" -> [w753]
                  tunnel: w740 -> [w745]
                  tunnel: [w744] -> w739 mode=indexing
                  tunnel: w733 -> [w743]
                  tunnel: [w741] -> w732 mode=indexing
                  i -> [w752]
                  n396 = Multiply(x=w743, y=w752) -> (x*y=w751:dbl)
                  n397 = Add(x=w753, y=w751) -> (x+y=w748:dbl)
                  n398 = local read "Scan axis"() -> (w742:bool)
                  n399 = local read "AO1"() -> (w750:dbl)
                  n400 = local read "AO2"() -> (w749:dbl)
                  n401 = Select(t=w748, s=w742, f=w750) -> (s? t:f=w747:dbl)
                  n402 = Select(t=w749, s=w742, f=w748) -> (s? t:f=w746:dbl)
                  n403 = flat-sequence {
                    tunnel: w747 -> [w757]
                    tunnel: w746 -> [w756]
                    tunnel: w745 -> [w754]
                    tunnel: [w767] -> w744
                    tunnel: [w766] -> w741
                    frame #0 {
                      w760 = 10.0 ("y")
                      w755 = 32767.0 ("y")
                      n404 = Multiply(x=w757, y=w755) -> (x*y=w763:dbl)
                      n405 = Multiply(x=w756, y=w755) -> (x*y=w761:dbl)
                      n406 = Divide(x=w763, y=w760) -> (x/y=w764:dbl)
                      n407 = Divide(x=w761, y=w760) -> (x/y=w762:dbl)
                      n408 = To Word Integer(number=w764) -> (16bit integer=w758:i16)
                      n409 = To Word Integer(number=w762) -> (16bit integer=w759:i16)
                      n410 = xnode "Read/Write Control"("FPGA VI Reference In"=w754, "AO1 (Y)"=w758, "AO2 (X)"=w759) -> ()  [unwired: 1 in, 2 out]
                    }
                    frame #1 {
                      n411 = Wait (ms)(milliseconds to wait="DAQ Delay (ms)") -> ()  [unwired: 1 out]
                    }
                    frame #2 {
                      n412 = local read "Slow mean"() -> (w767:dbl)
                      n413 = local read "Sigma"() -> (w766:dbl)
                    }
                  }
                }
                n414 = Bundle("Begin (V)"="Begin (V)", w733, w739) -> (→"MCL Scan":cluster{"Begin (V)":dbl, dbl, dbl[]})  [unwired: 1 out]
                n415 = Bundle("Begin (V)"="Begin (V)", w733, w732) -> (→"MCL Scan 2":cluster{"Begin (V)":dbl, dbl, dbl[]})  [unwired: 1 out]
              }
            }
          }
        }
        n416 = local read "Stop All"() -> (w677:bool)
        n417 = node-c288() -> ()  [unwired: 2 out]
      }
      n418 = node-c288(w674) -> ()  [unwired: 1 out]
    }
    frame Disabled {
    }
  }
  n419 = node-c288(2 ("Processor")) -> (w54:T25)  [unwired: 3 in]
  n420 = timed-loop "Control parameters (event loop)" {
    tunnel: w61 -> [w773]
    shift-right: [w772] -> _
    shift-left: errorcluster {"status"=FALSE, "code"=0, "source"=""} ("error out") -> [w771]
    tunnel: [w770] -> w73
    timing: w54 -> [_]
    timing-out: [_] -> w53
    stop <- w770 stop-if-true
    n421 = node-c288() -> ()  [unwired: 1 in, 1 out]
    n422 = event shown="[0] \"AI Count (ticks)\", \"Sets to FIFO (Traps)\", \"Save ave N\", \"FPGA Ave.\", \"# Samples/channel\", \"N sets to save\": Value Change" {
      selector: _ -> [_ _ _ _ _ _ _ _ _ _ _ _ _ _ _ _ _ _ _ _ _ _ _ _ _ _ _ _ _ _ _ _ _ _ _ _ _ _ _ _ _ _ _ _ _ _ _ _ _ _ _ _ _ _ _ _ _ _ _ _ _ _]
      dyn-events: _ -> [_ _ _ _ _ _ _ _ _ _ _ _ _ _ _ _ _ _ _ _ _ _ _ _ _ _ _ _ _ _ _ _ _ _ _ _ _ _ _ _ _ _ _ _ _ _ _ _ _ _ _ _ _ _ _ _ _ _ _ _ _ _]
      timeout: _ -> [_ _ _ _ _ _ _ _ _ _ _ _ _ _ _ _ _ _ _ _ _ _ _ _ _ _ _ _ _ _ _ _ _ _ _ _ _ _ _ _ _ _ _ _ _ _ _ _ _ _ _ _ _ _ _ _ _ _ _ _ _ _]
      tunnel: w773 -> [w814 _ _ _ w851 _ w869 w875 _ _ _ _ w952 _ _ w996 w1002 w1006 w1011 w1047 w1065 w1072 w1090 w1101 w1112 w1123 w1134 w1145 w1163 w1169 w1263 _ w1275 w1313 _ w1383 w1388 w1392 w1403 w1408 w1432 _ w1440 _ _ _ _ _ w1576 _ w1593 w1608 w1634 w1637 w1660 w1720 _ w1737 w1740 _ _ _]
      tunnel: [w813 _ _ _ w841 _ _ w874 _ _ w917 _ w932 _ _ w995 w998 w1005 w1008 w1046 w1063 w1071 w1084 w1095 w1106 w1117 w1128 w1139 w1161 w1168 w1261 _ w1273 w1311 _ _ w1386 w1390 w1393 w1406 w1430 _ w1438 _ _ _ _ _ w1574 _ _ _ _ _ _ _ _ _ _ _ _ _] -> w772
      tunnel: w771 -> [w812 _ _ _ w850 _ _ w873 _ _ w917 _ w951 _ _ w994 w997 w1004 w1007 w1045 w1064 w1070 w1089 w1100 w1111 w1122 w1133 w1144 w1162 w1167 w1262 _ w1274 w1312 _ _ w1387 w1391 w1402 w1407 w1431 _ w1439 _ _ _ _ _ w1575 _ w1592 w1607 w1633 w1636 w1661 w1719 _ w1736 _ _ _ _]
      tunnel: [_ _ _ _ _ _ _ _ _ _ w916 _ _ _ _ _ _ _ _ _ _ _ _ _ _ _ _ _ _ _ _ _ _ _ _ _ _ _ _ _ _ _ _ _ _ _ _ _ _ _ _ _ _ _ _ _ _ _ _ _ _ _] -> w770
      tunnel: [_ _ _ _ _ _ _ _ "Round T1 X" _ _ _ _ _ _ _ _ _ _ _ _ _ _ _ _ _ _ _ _ _ _ _ _ _ _ _ _ _ _ _ _ _ _ _ _ _ _ _ _ _ _ _ _ _ _ _ _ _ _ _ _ _] -> _
      tunnel: [_ _ _ "Adjust Scale\nto Mean" _ _ _ _ _ _ _ _ _ _ _ _ _ _ _ _ _ _ _ _ _ _ _ _ _ _ _ _ _ _ _ _ _ _ _ _ _ _ _ _ _ _ _ _ _ _ _ _ _ _ _ "Set SP to Reading" _ _ _ _ _ _] -> _
      tunnel: [_ _ _ _ _ _ _ _ _ "Round T2 X" _ "Delayed Interlace Start" _ _ _ _ _ _ _ _ _ _ _ _ _ _ _ _ _ _ _ _ _ _ _ _ _ _ _ _ _ _ _ _ _ _ _ _ _ _ _ _ _ _ _ _ _ _ _ _ _ _] -> _
      event "AI Count (ticks)", "Sets to FIFO (Traps)", "Save ave N", "FPGA Ave.", "# Samples/channel", "N sets to save": Value Change {
        # "So that if 'Save ave N' is updated, the AOD scanning code updates too."
        n423 = event-data() -> ()  [unwired: 6 out]
        n424 = local read "AI Count (ticks)"() -> (w795:u32)
        n425 = Unbundle By Name("Sets to FIFO (Traps)") -> ("Set 1"=w778:bool, "Set 2"=w777:bool, "Set 3"=w776:bool)
        n426 = Boolean To (0,1)(Boolean="Sets to FIFO (Traps)") -> (0, 1=w804:cluster{"Set 1":i16, "Set 2":i16, "Set 3":i16})
        n427 = xnode "Read/Write Control"("FPGA VI Reference In"=w814, "error in"=w812, "ai count"=w795, "Set 1"=w778, "Set 2"=w777, "Set 3"=w776, "N of AI1 Int Acq Sets"="N Acq Sets (Traps + Fl.)") -> ("error out"=w813:errorcluster)  [unwired: 1 out]
        n428 = Cluster To Array(cluster=w804) -> (array=w803:i16[])
        n429 = To Unsigned Long Integer(number=w803) -> (unsigned 32bit integer=w784:u32[])
        n430 = local read "Scan steps (AOD)"() -> (w805:u64)
        n431 = Multiply(x=w795, y="N Acq Sets (Traps + Fl.)") -> (x*y=w793:u32)
        n432 = Divide(x=40000000.0, y=w795) -> (x/y=w787:dbl)
        "AI rate (Hz)" <- w787
        "Ave. Rate (Hz)" <- w787
        n433 = Add Array Elements(numeric array=w784) -> (sum=w796:u32)
        "Trap Sets" <- w796
        n434 = Reciprocal(x=w787) -> (1/x=→"Ave. Period (s)":dbl)
        n435 = property on="Scan steps (AOD)" class="DigNum (strict)"("Val(Sgnl)"=w805) -> ()  [unwired: 2 in, 2 out]
        n436 = Divide(x=w787, y="N Acq Sets (Traps + Fl.)") -> (x/y=w809:dbl)
        "Data Rate (Hz)" <- w809
        n437 = Reciprocal(x=w809) -> (1/x=→"Data Period (s)":dbl)
        n438 = local read "Save ave N"() -> (w808:dbl)
        n439 = Divide(x=w809, y=w808) -> (x/y=w807:dbl)
        "Save Data Rate (Hz)" <- w807
        n440 = Reciprocal(x=w807) -> (1/x=→"Save Data Period (s)":dbl)
        n441 = Multiply(x=w793, y="# Samples/trap") -> (x*y=w791:u32)
        "Counts/DMA" <- w791
        n442 = property on="Trap Disp. Downsample" class="DigNum (strict)"("Maximum"="# Samples/trap") -> ()  [unwired: 2 in, 2 out]
        n443 = Multiply(x=w796, y="# Samples/trap") -> (x*y=w785:u32)
        "# Samples/channel" <- w785
        n444 = Multiply(x=w785, y=u32 8) -> (x*y=→"Trap AI Elements/DMA read":u32)
        n445 = local read "APD Int. Count"() -> (w792:u32)
        n446 = Multiply(x=w785, y=u32 3) -> (x*y=→"Trap Pos Elements/DMA read":u32)
        n447 = Divide(x=w791, y=w792) -> (x/y=w782:dbl)
        "APD Samples/FIFO Acq." <- w782
        n448 = Divide(x=w791, y=40000000.0) -> (x/y=w789:dbl)
        "DMA Update Period (s)" <- w789
        n449 = Multiply(x=2.0, y=w782) -> (x*y=→"APD Elements/DMA read":dbl)
        n450 = property on="APD Disp. Downsample" class="DigNum (strict)"("Maximum"=w782) -> ()  [unwired: 2 in, 2 out]
        n451 = local read "N sets to save"() -> (w801:u32)
        n452 = Multiply(x=w789, y=w801) -> (x*y=→"Total Time (s)":dbl)
        "FPGA Averaging" <- FALSE ("FPGA Averaging")
      }
      event "Rescale on Mean": Value Change {
        n453 = event-data() -> ()  [unwired: 7 out]
        n454 = And(x=FALSE, y="Rescale on Mean") -> (x .and. y?=w816:bool)
        n455 = local write "Rescale on Mean"(w816) -> ()
        n456 = local read "Bead Mean (nm)"() -> (w821:dbl)
        n457 = Add(x="Amplitude (nm)", y=w821) -> (x+y=w819:dbl)
        n458 = Subtract(x=w821, y="Amplitude (nm)") -> (x-y=w818:dbl)
        n459 = property on="Bead Separation" class="WFChart (strict)"("YScale.Minimum"=w818) -> ()  [unwired: 2 in, 2 out]
        n460 = property on="Bead Separation" class="WFChart (strict)"("YScale.Maximum"=w819) -> ()  [unwired: 2 in, 2 out]
      }
      event "Detector Type": Value Change {
        n461 = event-data() -> ()  [unwired: 7 out]
        n462 = local read "AI labels"() -> (w822:string[])
        n463 = property on="High Res. Display" class="Ring (strict)"("Strings []"=w822) -> ()  [unwired: 2 in, 2 out]
        n464 = Build Array (concatenate)(w822, "none") -> (w823:string[])
        n465 = property on="FFT 1 Choice 1" class="Ring (strict)"("Strings []"=w823) -> ()  [unwired: 2 in, 2 out]
        n466 = property on="FFT 1 Choice 2" class="Ring (strict)"("Strings []"=w823) -> ()  [unwired: 2 in, 2 out]
        n467 = property on="FFT 2 Choice 1" class="Ring (strict)"("Strings []"=w823) -> ()  [unwired: 2 in, 2 out]
        n468 = property on="FFT 2 Choice 2" class="Ring (strict)"("Strings []"=w823) -> ()  [unwired: 2 in, 2 out]
        n469 = Bundle("APD 1", "APD 2") -> (w826:cluster{string, string})  [unwired: 1 out]
        n470 = Cluster To Array(cluster=w826) -> (array=w824:string[])
        n471 = Build Array (concatenate)(w824, w823) -> (w828:string[])
        n472 = Array Size(array=w828) -> (size(s)=w829:i32)
        n473 = property on="Signals to Plot" class="LstBox (strict)"("Item Names"=w828) -> ()  [unwired: 2 in, 2 out]
        n474 = property on="Signals to Plot" class="LstBox (strict)"("Number of Rows"=w829) -> ()  [unwired: 2 in, 2 out]
        n475 = property on="All Signals" class="WFChart (strict)"("LegNumRows"=w829) -> ()  [unwired: 2 in, 2 out]
      }
      event "Adjust Scale\nto Mean": Value Change {
        n476 = event-data() -> ()  [unwired: 7 out]
        n477 = local read "APD 1 Rate (Hz)"() -> (w838:dbl)
        n478 = Multiply(x=1000.0, y="Above (kHz)") -> (x*y=w836:dbl)
        n479 = Multiply(x=1000.0, y="Below (kHz)") -> (x*y=w834:dbl)
        n480 = Add(x=w836, y=w838) -> (x+y=w831:dbl)
        n481 = Subtract(x=w838, y=w834) -> (x-y=w832:dbl)
